vi "regionTester.vi"() -> ()   [LabVIEW 2013]
panel:
  out "Motor Output":dbl
  in  "DownLimit":bool
  in  "Down2":bool
  in  "Center":bool
  in  "Up2":bool
  in  "UpLimit":bool
  in  "Axis":dbl
  out "Region":dbl
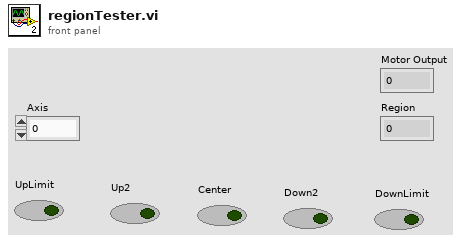
[diagram p1: front panel]
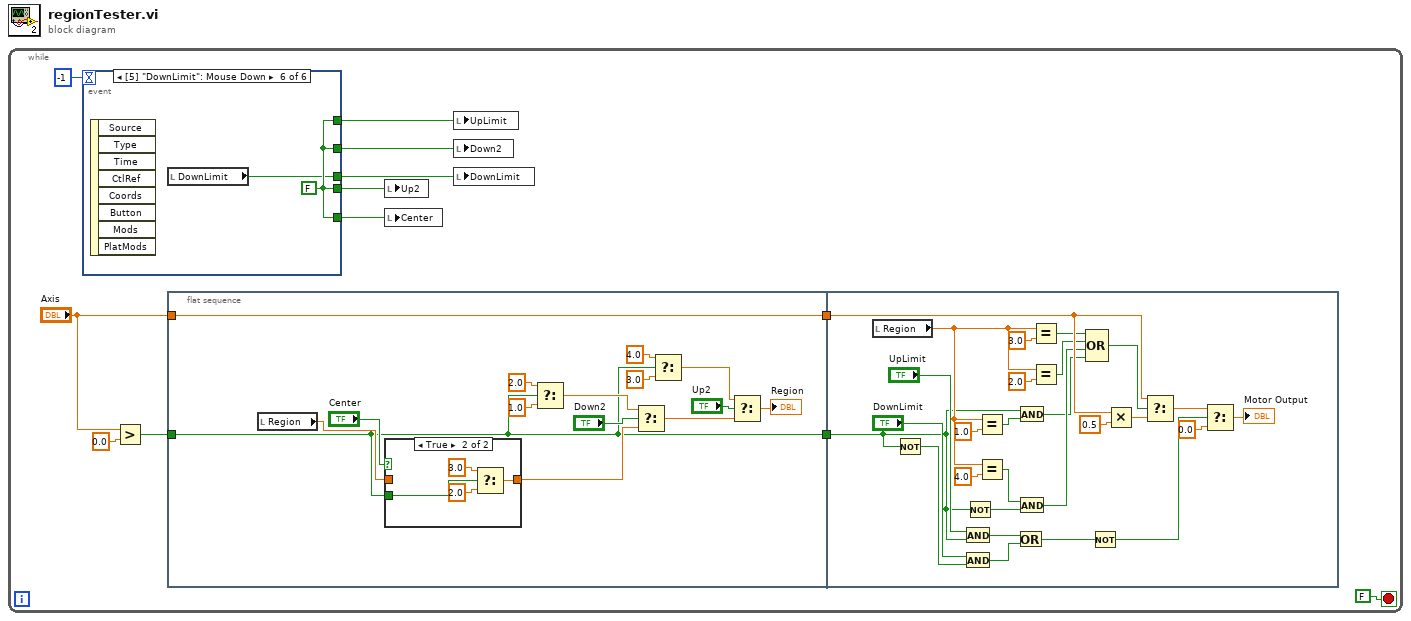
[diagram p0: block diagram]
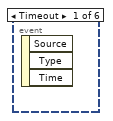
[diagram p2: hidden frame]
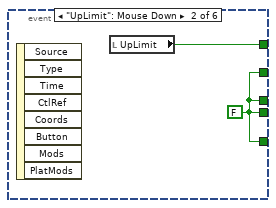
[diagram p3: hidden frame]
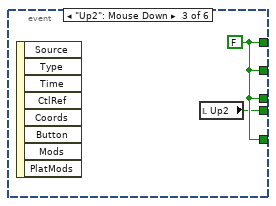
[diagram p4: hidden frame]
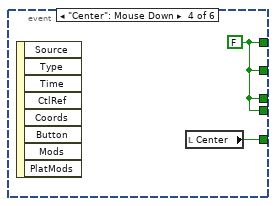
[diagram p5: hidden frame]
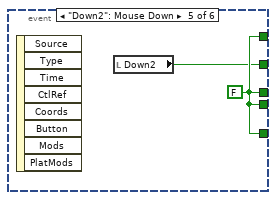
[diagram p6: hidden frame]
diagram:
  n1 = while {
    stop <- FALSE stop-if-true
    n2 = event shown="[5] \"DownLimit\": Mouse Down" {
      selector: _ -> [_ _ _ _ _ _]
      dyn-events: _ -> [_ _ _ _ _ _]
      timeout: -1 -> [_ _ _ _ _ _]
      tunnel: [_ w13 w16 w18 w20 w22] -> w5
      tunnel: [_ w14 w15 w18 w20 w22] -> w4
      tunnel: [_ w14 w16 w17 w20 w22] -> w3
      tunnel: [_ w14 w16 w18 w19 w22] -> w2
      tunnel: [_ w14 w16 w18 w20 w21] -> w1
      event Timeout {
        n3 = event-data() -> ()  [unwired: 1 in, 3 out]
      }
      event "UpLimit": Mouse Down {
        w14 = FALSE
        n4 = event-data() -> ()  [unwired: 1 in, 8 out]
        n5 = local read "UpLimit"() -> (w13:bool)
      }
      event "Up2": Mouse Down {
        w16 = FALSE
        n6 = event-data() -> ()  [unwired: 1 in, 8 out]
        n7 = local read "Up2"() -> (w15:bool)
      }
      event "Center": Mouse Down {
        w18 = FALSE
        n8 = event-data() -> ()  [unwired: 1 in, 8 out]
        n9 = local read "Center"() -> (w17:bool)
      }
      event "Down2": Mouse Down {
        w20 = FALSE
        n10 = event-data() -> ()  [unwired: 1 in, 8 out]
        n11 = local read "Down2"() -> (w19:bool)
      }
      event "DownLimit": Mouse Down {
        w22 = FALSE
        n12 = event-data() -> ()  [unwired: 1 in, 8 out]
        n13 = local read "DownLimit"() -> (w21:bool)
      }
    }
    n14 = Greater?(x="Axis", y=0.0) -> (0:w7:bool)
    n15 = flat-sequence {
      tunnel: "Axis" -> [w37]
      tunnel: w7 -> [w23]
      tunnel: [w23] -> w9
      tunnel: [w37] -> w8
      tunnel: w9 -> [w49]
      tunnel: w8 -> [w48]
      frame #0 {
        n16 = local read "Region"() -> (w24:dbl)
        n17 = case shown="True" "Center" {
          tunnel: w23 -> [_ w42]
          tunnel: [w38 w39] -> w32
          tunnel: w24 -> [w38 _]
          frame False {
          }
          frame True {
            n18 = Select(t=3.0, s=w42, f=2.0) -> (s? t:f=w39:dbl)
          }
        }
        n19 = Select(t=2.0, s=w23, f=1.0) -> (s? t:f=w28:dbl)
        n20 = Select(t=w28, s="Down2", f=w32) -> (s? t:f=w31:dbl)
        n21 = Select(t=4.0, s=w23, f=3.0) -> (s? t:f=w25:dbl)
        n22 = Select(t=w25, s="Up2", f=w31) -> (s? t:f=→"Region":dbl)
      }
      frame #1 {
        n23 = local read "Region"() -> (w50:dbl)
        n24 = Not(x=w49) -> (.not. x?=w56:bool)
        n25 = And(x="UpLimit", y=w49) -> (x .and. y?=w55:bool)
        n26 = And(x="DownLimit", y=w56) -> (x .and. y?=w54:bool)
        n27 = Not(x=w49) -> (.not. x?=w60:bool)
        n28 = Equal?(x=w50, y=1.0) -> (x = y?=w65:bool)
        n29 = Equal?(x=w50, y=4.0) -> (x = y?=w61:bool)
        n30 = Or(x=w55, y=w54) -> (x .or. y?=w52:bool)
        n31 = And(x=w49, y=w65) -> (x .and. y?=w44:bool)
        n32 = And(x=w61, y=w60) -> (x .and. y?=w45:bool)
        n33 = Equal?(x=w50, y=3.0) -> (x = y?=w47:bool)
        n34 = Equal?(x=w50, y=2.0) -> (x = y?=w46:bool)
        n35 = Compound Arithmetic op=OR(w47, w46, w45, w44) -> (w43:bool)
        n36 = Not(x=w52) -> (.not. x?=w51:bool)
        n37 = Multiply(x=w48, y=0.5) -> (x*y=w59:dbl)
        n38 = Select(t=w48, s=w43, f=w59) -> (s? t:f=w57:dbl)
        n39 = Select(t=w57, s=w51, f=0.0) -> (s? t:f=→"Motor Output":dbl)
      }
    }
    n40 = local write "Up2"(w4) -> ()
    n41 = local write "Center"(w3) -> ()
    n42 = local write "UpLimit"(w5) -> ()
    n43 = local write "Down2"(w2) -> ()
    n44 = local write "DownLimit"(w1) -> ()
  }
